vi "MainVI.vi"() -> ()   [LabVIEW 2021]
uses:
  <vilib>/Instr/_visa.llb/VISA Find Search Mode.ctl
  <vilib>/Instr/_visa.llb/VISA Configure Serial Port (Instr).vi
panel:
  out "No Error":bool[](array[boolean])
  out "Error":bool[](array[boolean])
  in  "error in (no error)":errorcluster
  out "error out":errorcluster
  out "VISA resource name out":refnum<visa-resource-name>
  in  "Number of lines in Output":i32
  out "find list":string[](array[string])
  in  "Write":bool
  in  "Stop":bool
  in  "Read":bool
  in  "Command":string="*IDN?"
  out "Response":string
  in  "Read Count":u32=1000
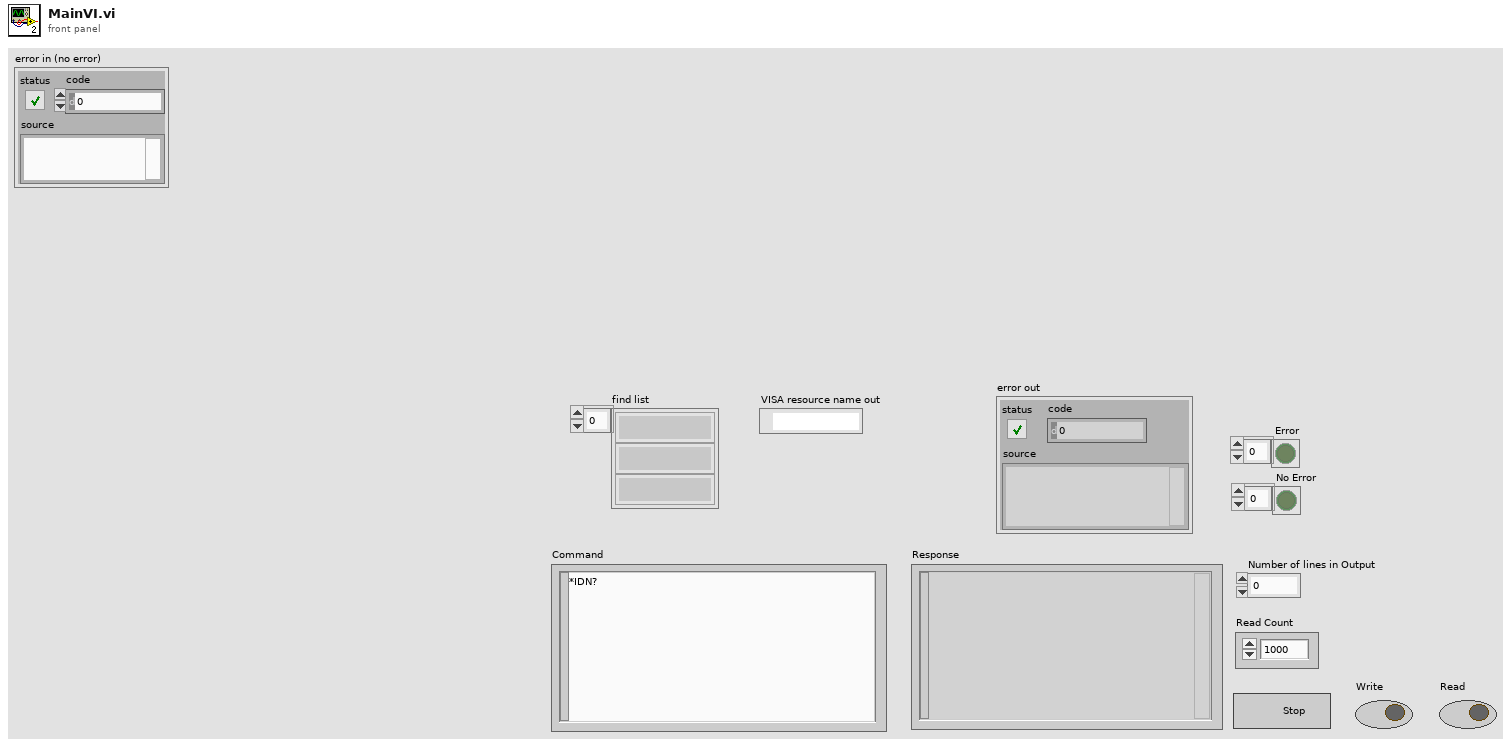
[diagram p1: front panel]
types:
  T1 = typedef "VISA Find Search Mode.ctl" = u32
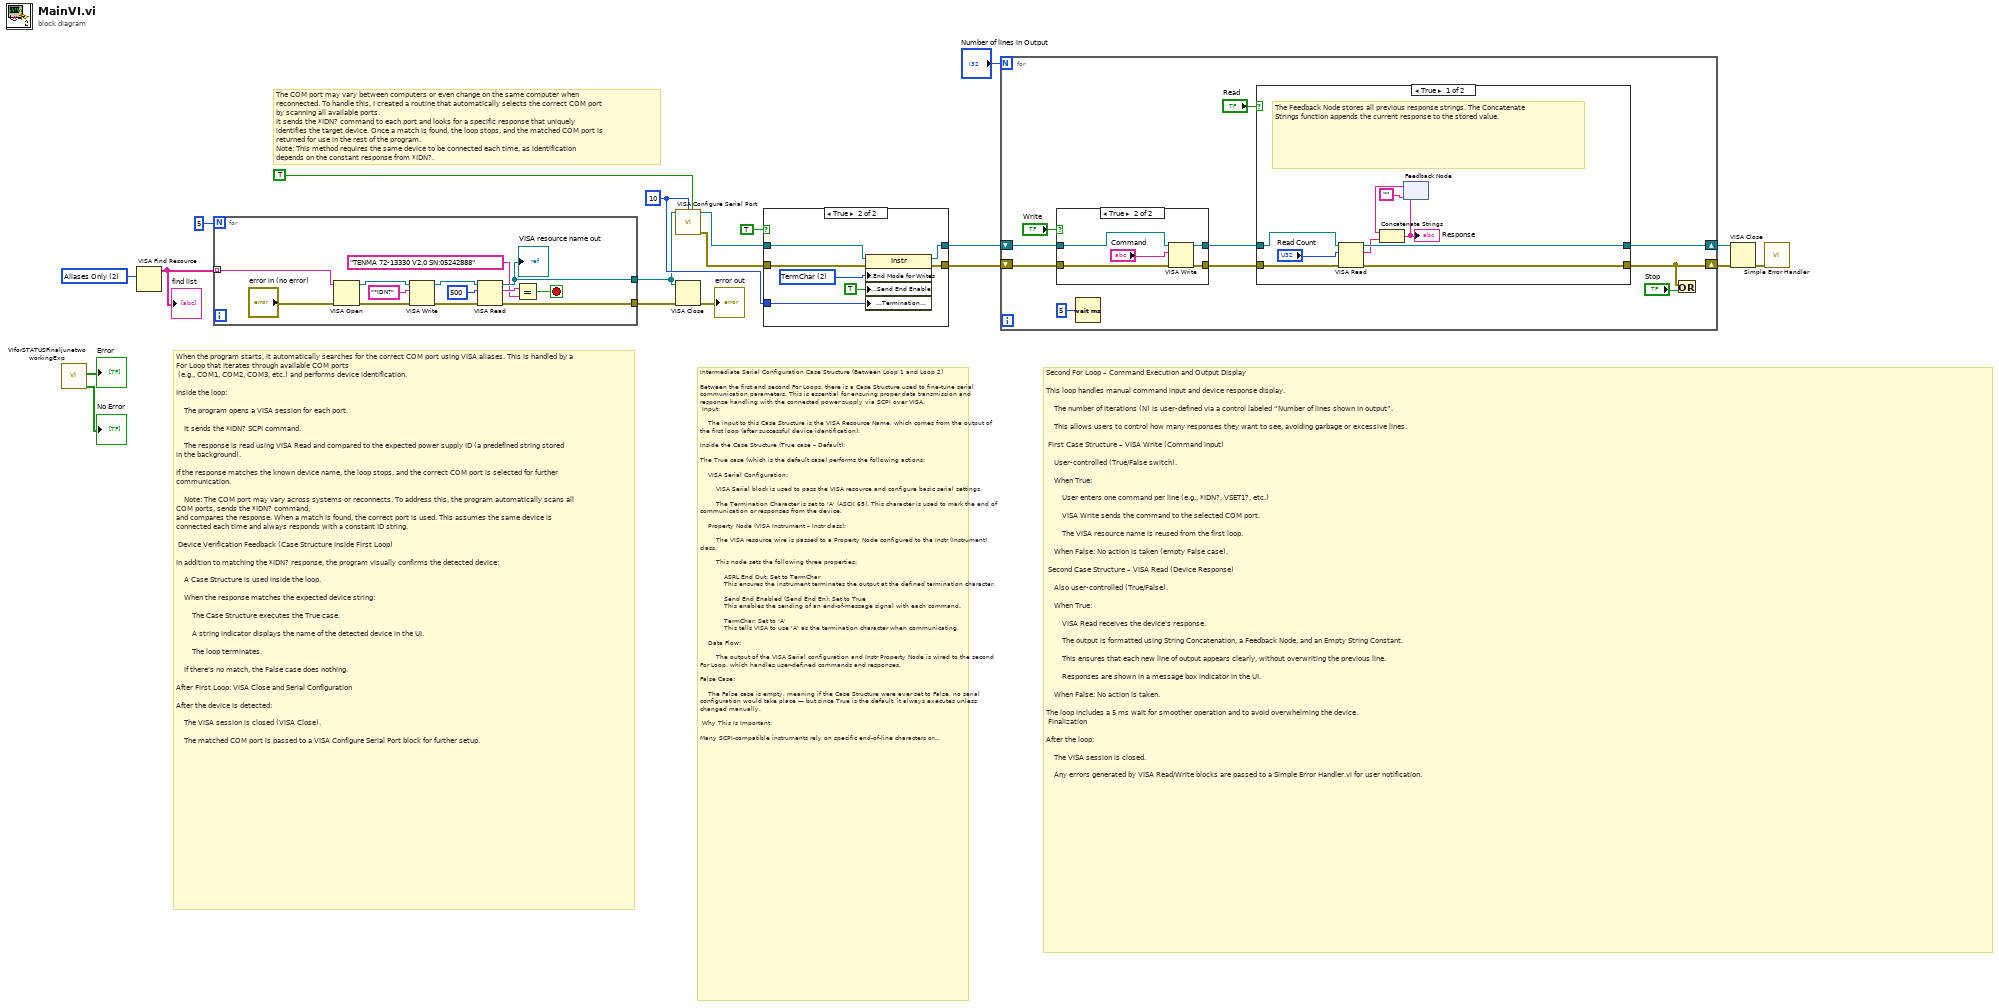
[diagram p0: block diagram]
diagram:
  w12 = u8 10 ("Termination Character")
  w5 = T1 2 items=["Canonical Names Only"=0, "Aliases Only"=2, "Include Matching Aliases"=3, "Include All Aliases"=4] ("Search Mode")
  # "Second For Loop – Command Execution and Output Display\n\nThis loop handles manual command input and device response display.\n\n    The number of iterations (N) is user-defined via a control labeled “Number of lines shown in output”.\n\n    This allows users to control how many responses they want to see, avoiding garbage or excessive lines.\n\n First Case Structure – VISA Write (Command Input)\n\n    User-controlled (True/False switch).\n\n    When True:\n\n        User enters one command per line (e.g., *IDN?, VSET1?, etc.)\n\n        VISA Write sends the command to the selected COM port.\n\n        The VISA resource name is reused from the first loop.\n\n    When False: No action is taken (empty False case).\n\n Second Case Structure – VISA Read (Device Response)\n\n    Also user-controlled (True/False).\n\n    When True:\n\n        VISA Read receives the device's response.\n\n        The output is formatted using String Concatenation, a Feedback Node, and an Empty String Constant.\n\n        This ensures that each new line of output appears clearly, without overwriting the previous line.\n\n        Responses are shown in a message box indicator in the UI.\n\n    When False: No action is taken.\n\nThe loop includes a 5 ms wait for smoother operation and to avoid overwhelming the device.\n Finalization\n\nAfter the loop:\n\n    The VISA session is closed.\n\n    Any errors generated by VISA Read/Write blocks are passed to a Simple Error Handler.vi for user notification."
  # "Intermediate Serial Configuration Case Structure (Between Loop 1 and Loop 2)\n\nBetween the first and second For Loops, there is a Case Structure used to fine-tune serial communication parameters. This is essential for ensuring proper data transmission and response handling with the connected power supply via SCPI over VISA.\n Input:\n\n    The input to this Case Structure is the VISA Resource Name, which comes from the output of the first loop (after successful device identification).\n\nInside the Case Structure (True case – Default):\n\nThe True case (which is the default case) performs the following actions:\n\n    VISA Serial Configuration:\n\n        VISA Serial block is used to pass the VISA resource and configure basic serial settings.\n\n        The Termination Character is set to 'A' (ASCII 65). This character is used to mark the end of communication or responses from the device.\n\n    Property Node (VISA Instrument – Instr class):\n\n        The VISA resource wire is passed to a Property Node configured to the Instr (Instrument) class.\n\n        This node sets the following three properties:\n\n            ASRL End Out: Set to TermChar\n            This ensures the instrument terminates the output at the defined termination character.\n\n            Send End Enabled (Send End En): Set to True\n            This enables the sending of an end-of-message signal with each command.\n\n            TermChar: Set to 'A'\n            This tells VISA to use 'A' as the termination character when communicating.\n\n    Data Flow:\n\n        The output of the VISA Serial configuration and Instr Property Node is wired to the second For Loop, which handles user-defined commands and responses.\n\nFalse Case:\n\n    The False case is empty, meaning if the Case Structure were ever set to False, no serial configuration would take place — but since True is the default, it always executes unless changed manually.\n\n Why This Is Important:\n\nMany SCPI-compatible instruments rely on specific end-of-line characters or termination protocols to know when a command or response is complete. This block ensures:\n\n    The commands sent are properly terminated.\n\n    The device's responses are interpreted correctly.\n\n    Compatibility is maintained regardless of the underlying COM port or system."
  # "When the program starts, it automatically searches for the correct COM port using VISA aliases. This is handled by a For Loop that iterates through available COM ports\n (e.g., COM1, COM2, COM3, etc.) and performs device identification.\n\nInside the loop:\n\n    The program opens a VISA session for each port.\n\n    It sends the *IDN? SCPI command.\n\n    The response is read using VISA Read and compared to the expected power supply ID (a predefined string stored in the background).\n\nIf the response matches the known device name, the loop stops, and the correct COM port is selected for further communication.\n\n    Note: The COM port may vary across systems or reconnects. To address this, the program automatically scans all COM ports, sends the *IDN? command, \nand compares the response. When a match is found, the correct port is used. This assumes the same device is connected each time and always responds with a constant ID string.\n\n Device Verification Feedback (Case Structure Inside First Loop)\n\nIn addition to matching the *IDN? response, the program visually confirms the detected device:\n\n    A Case Structure is used inside the loop.\n\n    When the response matches the expected device string:\n\n        The Case Structure executes the True case.\n\n        A string indicator displays the name of the detected device in the UI.\n\n        The loop terminates.\n\n    If there's no match, the False case does nothing.\n\nAfter First Loop: VISA Close and Serial Configuration\n\nAfter the device is detected:\n\n    The VISA session is closed (VISA Close).\n\n    The matched COM port is passed to a VISA Configure Serial Port block for further setup."
  # "The COM port may vary between computers or even change on the same computer when reconnected. To handle this, I created a routine that automatically selects the correct COM port by scanning all available ports.\nIt sends the *IDN? command to each port and looks for a specific response that uniquely identifies the target device. Once a match is found, the loop stops, and the matched COM port is returned for use in the rest of the program.\nNote: This method requires the same device to be connected each time, as identification depends on the constant response from *IDN?."
  n1 = call "VIforSTATUSFinaljunetwoworkingExp.vi"() -> ("Error 2"=→"No Error":bool[], "Error"=→"Error":bool[])  [unwired: 8 in, 2 out]
  n2 = VISA Find Resource(10:w5) -> (3:w8:string[])  [unwired: 2 in, 2 out]
  "find list" <- w8
  n3 = for {
    N: 5 -> [_]
    tunnel: w8 -> [w32] mode=indexing
    tunnel: [w25] -> w7
    tunnel: [w24] -> w6
    stop <- w21 stop-if-true
    n4 = VISA Open(error in (no error)="error in (no error)", VISA resource name=w32) -> (VISA resource name=w31:refnum<visa-resource-name>, error out=w29:errorcluster)  [unwired: 3 in]
    n5 = VISA Write(VISA resource name=w31, write buffer="*IDN?", error in (no error)=w29) -> (VISA resource name out=w28:refnum<visa-resource-name>, error out=w26:errorcluster)  [unwired: 1 out]
    n6 = VISA Read(VISA resource name=w28, byte count=u32 500, error in (no error)=w26) -> (VISA resource name out=w24:refnum<visa-resource-name>, read buffer=w23:string, error out=w25:errorcluster)  [unwired: 1 out]
    "VISA resource name out" <- w24
    n7 = Equal?(x=w23, y="TENMA 72-13330 V2.0 SN:05242888") -> (x = y?=w21:bool)
  }
  n8 = call-poly "VISA Configure Serial Port"("VISA resource name"=w6, "termination char\n(0xA = '\\n' = LF)"=w12, "Enable Termination\nChar (T)"=TRUE ("End Read on Termination Character?")) -> ("VISA resource name out"=w11:refnum<visa-resource-name>, "error out"=w10:errorcluster)  [unwired: 7 in, 4 out]
  n9 = VISA Close(VISA resource name=w6, error in (no error)=w7) -> (error out=→"error out":errorcluster)
  n10 = case shown="True" TRUE ("End Write on Termination Character?") {
    tunnel: w11 -> [w33 w41]
    tunnel: w10 -> [w34 w40]
    tunnel: [w33 w39] -> w14
    tunnel: [w34 w38] -> w15
    tunnel: w12 -> [_ w36]
    frame False {
    }
    frame True {
      w37 = u16 2 items=["None", "LastBit", "TermChar", "Break"] ("Serial Settings:Serial End Mode for Writes")
      n11 = property class="Instr"(reference=w41, error in=w40, "Serial Settings:End Mode for Writes"=w37, "Message Based Settings:Send End Enable"=TRUE, "Message Based Settings:Termination Character"=w36) -> (reference out=w39:refnum<visa-resource-name>, error out=w38:errorcluster)
    }
  }
  n12 = for {
    N: "Number of lines in Output" -> [_]
    shift-right: [w51] -> w17
    shift-left: w15 -> [w49]
    shift-right: [w50] -> w16
    shift-left: w14 -> [w48]
    n13 = case shown="True" "Write" {
      tunnel: w48 -> [w53 w57]
      tunnel: w49 -> [w52 w56]
      tunnel: [w53 w55] -> w47
      tunnel: [w52 w54] -> w46
      frame False {
      }
      frame True {
        n14 = VISA Write(VISA resource name=w57, write buffer="Command", error in (no error)=w56) -> (VISA resource name out=w55:refnum<visa-resource-name>, error out=w54:errorcluster)  [unwired: 1 out]
      }
    }
    n15 = Wait (ms)(milliseconds to wait=u32 5) -> ()  [unwired: 1 out]
    n16 = case shown="True" "Read" {
      tunnel: [w65 w69] -> w50
      tunnel: w47 -> [w67 w69]
      tunnel: [w63 w68] -> w51
      tunnel: w46 -> [w66 w68]
      frame True {
        # "The Feedback Node stores all previous response strings. The Concatenate Strings function appends the current response to the stored value."
        n17 = VISA Read(VISA resource name=w67, byte count="Read Count", error in (no error)=w66) -> (VISA resource name out=w65:refnum<visa-resource-name>, read buffer=w62:string, error out=w63:errorcluster)  [unwired: 1 out]
        n18 = feedback #1("") -> (w61:string)
        n19 = Concatenate Strings(w61, w62) -> (w60:string)
        "Response" <- w60
        n20 = feedback-in #1(w60) -> ()
      }
      frame False {
      }
    }
    n21 = Or(x=w51, y="Stop") -> ()  [unwired: 1 out]
  }
  n22 = VISA Close(VISA resource name=w16, error in (no error)=w17) -> (error out=w18:errorcluster)
  n23 = call <vilib>:"Simple Error Handler.vi"("error in (no error)"=w18) -> ()  [unwired: 1 in, 8 out]
